vi "intitialize RF synth boards on FPGA 12.5.vi"() -> ()   [LabVIEW 2013]
uses:
  <vilib>/Platform/TimedLoop/XDataNode/timing_clust.ctl
  <vilib>/Platform/TimedLoop/XDataNode/nitl_modes.ctl
  <vilib>/Platform/TimedLoop/XDataNode/wakeup.ctl
  <vilib>/rvi/eio/common/nirviEmuTemplateMethod_errors.vi
  <vilib>/rvi/Emulation/niFpgaSctlEmulationGetInTimedLoop.vi
  <vilib>/rvi/Emulation/niFpgaEmulationReportErrorSimple.vi
  <vilib>/rvi/Emulation/niFpgaGetClockAttributes.vi
  <vilib>/rvi/Emulation/niFpgaCriticalErrorInLSC.vi
  <vilib>/Platform/TimedLoop/XDataNode/XDataNode.xnode
  <vilib>/eio/EIONode/EIONode.xnode
  <vilib>/eio/EIOMethodNode/EIOMethodNode.xnode
  <vilib>/Platform/TimedLoop/XDataNode/XDNodeRunTimeDep.lvlib
panel:
  in  "OSK Bd 1":bool
  in  "Reset Bd 1":bool
  in  "PMODE":bool
  in  "RD":bool
  in  "Address":u8 format="%02x"
  in  "Data BD 1":u8 format="%08b"
  in  "Data BD 2":u8 format="%08b"
  in  "Update Data":bool
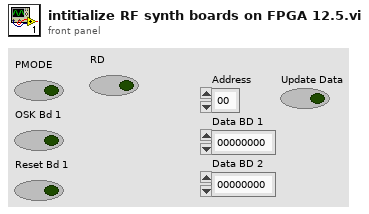
[diagram p1: front panel]
types:
  T1 = typedef "XDNodeRunTimeDep.lvlib/timing_clust.ctl" = cluster{"Expected End [f-1]":u64, "Actual End [f-1]":u64, "Finished Late? [f-1]":bool, "Expected End [i-1]":u64, "Actual End [i-1]":u64, "Finished Late? [i-1]":bool, "Expected Start [i]":u64, "Actual Start [i]":u64, "Expected Start [f]":u64, "Actual Start [f]":u64, "Source Name":string, "Structure Name":string, "Period":i64, "Deadline":i64, "Offset":i64, "Start":i64, "Priority":i32, "Timeout":i32, "Mode":T2, "Wakeup Reason":T3, "Error":errorcluster, "Source Type":string, "Secondary Source Type":string, "Global End Time":u64, "Global Start Time":u64, "Frame Duration":u64, "Iteration Duration":u64, "Assigned CPU":i32, "I/O Scan Engine Mode":u32}
  T2 = typedef "XDNodeRunTimeDep.lvlib/nitl_modes.ctl" = enum32{"No Change", "Process missed periods, maintain original phase", "Discard missed periods, maintain original phase", "Process missed periods, ignore original phase", "Discard missed periods, ignore original phase"}
  T3 = typedef "XDNodeRunTimeDep.lvlib/wakeup.ctl" = enum32{"Normal", "Aborted", "Asynchronous wakeup", "Timing source error", "Timed loop error", "Timeout"}
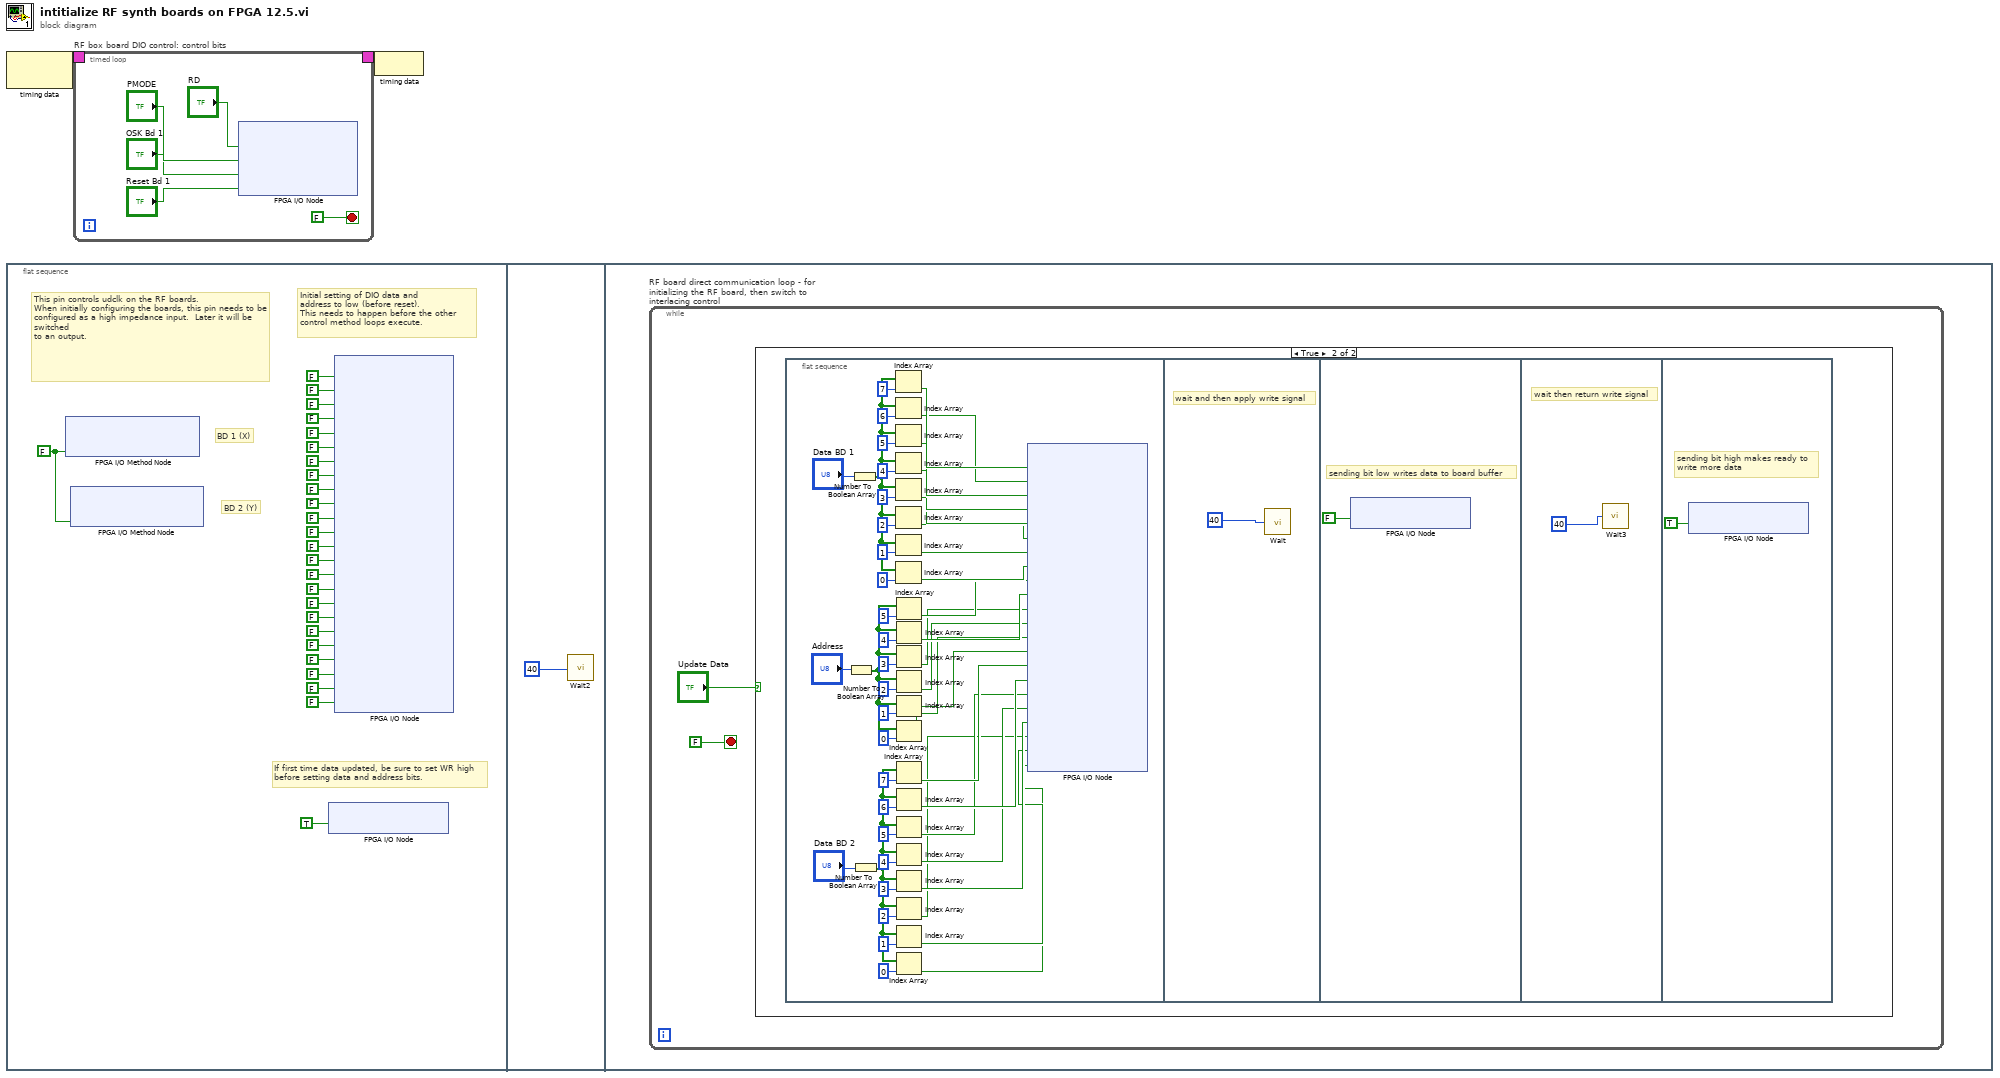
[diagram p0: block diagram]
diagram:
  n1 = node-c288() -> (w2:T1)  [unwired: 1 in]
  n2 = flat-sequence {
    frame #0 {
      w4 = FALSE ("Enable")
      # "If first time data updated, be sure to set WR high\nbefore setting data and address bits."
      # "BD 2 (Y)"
      # "BD 1 (X)"
      # "This pin controls udclk on the RF boards.\nWhen initially configuring the boards, this pin needs to be\nconfigured as a high impedance input.  Later it will be switched\nto an output."
      # "Initial setting of DIO data and \naddress to low (before reset).  \nThis needs to happen before the other\ncontrol method loops execute."
      n3 = xnode "FPGA I/O Method Node"("Enable"=w4) -> ()  [unwired: 1 in, 1 out]
      n4 = xnode "FPGA I/O Method Node"("Enable"=w4) -> ()  [unwired: 1 in, 1 out]
      n5 = xnode "FPGA I/O Node"("Connector1/DIO15"=TRUE) -> ()  [unwired: 1 in, 1 out]
      n6 = xnode "FPGA I/O Node"("Connector1/DIO0"=FALSE, "Connector1/DIO1"=FALSE, "Connector1/DIO2"=FALSE, "Connector1/DIO3"=FALSE, "Connector1/DIO4"=FALSE, "Connector1/DIO5"=FALSE, "Connector1/DIO6"=FALSE, "Connector1/DIO7"=FALSE, "Connector1/DIO8"=FALSE, "Connector1/DIO9"=FALSE, "Connector1/DIO10"=FALSE, "Connector1/DIO11"=FALSE, "Connector1/DIO12"=FALSE, "Connector1/DIO13"=FALSE, "Connector1/DIO15"=FALSE, "Connector1/DIO20"=FALSE, "Connector1/DIO21"=FALSE, "Connector1/DIO22"=FALSE, "Connector1/DIO23"=FALSE, "Connector1/DIO24"=FALSE, "Connector1/DIO25"=FALSE, "Connector1/DIO26"=FALSE, "Connector1/DIO27"=FALSE, "Connector1/DIO14"=FALSE) -> ()  [unwired: 24 in, 24 out]
    }
    frame #1 {
      n7 = call "Wait2"("Count(Ticks)"=u8 40 ("DO Delay 3 (Ticks)")) -> ()  [unwired: 1 out]
    }
    frame #2 {
      n8 = while "RF board direct communication loop - for initializing the RF board, then switch to interlacing control" {
        stop <- FALSE stop-if-true
        n9 = case shown="True" "Update Data" {
          frame False {
          }
          frame True {
            n10 = flat-sequence {
              frame #0 {
                n11 = Number To Boolean Array(number="Address") -> (Boolean array=w78:bool[])
                n12 = Number To Boolean Array(number="Data BD 1") -> (Boolean array=w79:bool[])
                n13 = Number To Boolean Array(number="Data BD 2") -> (Boolean array=w48:bool[])
                n14 = Index Array(array=w79, index=7) -> (element=w63:bool)
                n15 = Index Array(array=w79, index=6) -> (element=w62:bool)
                n16 = Index Array(array=w79, index=5) -> (element=w61:bool)
                n17 = Index Array(array=w79, index=4) -> (element=w60:bool)
                n18 = Index Array(array=w79, index=3) -> (element=w59:bool)
                n19 = Index Array(array=w79, index=2) -> (element=w58:bool)
                n20 = Index Array(array=w79, index=1) -> (element=w57:bool)
                n21 = Index Array(array=w79, index=0) -> (element=w56:bool)
                n22 = Index Array(array=w78, index=5) -> (element=w55:bool)
                n23 = Index Array(array=w78, index=4) -> (element=w54:bool)
                n24 = Index Array(array=w78, index=3) -> (element=w53:bool)
                n25 = Index Array(array=w78, index=2) -> (element=w52:bool)
                n26 = Index Array(array=w78, index=1) -> (element=w51:bool)
                n27 = Index Array(array=w78, index=0) -> (element=w50:bool)
                n28 = Index Array(array=w48, index=7) -> (element=w39:bool)
                n29 = Index Array(array=w48, index=6) -> (element=w38:bool)
                n30 = Index Array(array=w48, index=5) -> (element=w37:bool)
                n31 = Index Array(array=w48, index=4) -> (element=w36:bool)
                n32 = Index Array(array=w48, index=3) -> (element=w35:bool)
                n33 = Index Array(array=w48, index=2) -> (element=w34:bool)
                n34 = Index Array(array=w48, index=1) -> (element=w33:bool)
                n35 = Index Array(array=w48, index=0) -> (element=w32:bool)
                n36 = xnode "FPGA I/O Node"("Connector1/DIO0"=w63, "Connector1/DIO1"=w62, "Connector1/DIO2"=w61, "Connector1/DIO3"=w60, "Connector1/DIO4"=w59, "Connector1/DIO5"=w58, "Connector1/DIO6"=w57, "Connector1/DIO7"=w56, "Connector1/DIO8"=w55, "Connector1/DIO9"=w54, "Connector1/DIO10"=w53, "Connector1/DIO11"=w52, "Connector1/DIO12"=w51, "Connector1/DIO13"=w50, "Connector1/DIO20"=w39, "Connector1/DIO21"=w38, "Connector1/DIO22"=w37, "Connector1/DIO23"=w36, "Connector1/DIO24"=w35, "Connector1/DIO25"=w34, "Connector1/DIO26"=w33, "Connector1/DIO27"=w32) -> ()  [unwired: 22 in, 22 out]
              }
              frame #1 {
                # "wait and then apply write signal"
                n37 = call "Wait"("Count(Ticks)"=u8 40 ("DO Delay 1 (Ticks)")) -> ()  [unwired: 1 out]
              }
              frame #2 {
                # "sending bit low writes data to board buffer"
                n38 = xnode "FPGA I/O Node"("Connector1/DIO15"=FALSE) -> ()  [unwired: 1 in, 1 out]
              }
              frame #3 {
                # "wait then return write signal"
                n39 = call "Wait3"("Count(Ticks)"=u8 40 ("DO Delay 2 (Ticks)")) -> ()  [unwired: 1 out]
              }
              frame #4 {
                # "sending bit high makes ready to\nwrite more data"
                n40 = xnode "FPGA I/O Node"("Connector1/DIO15"=TRUE) -> ()  [unwired: 1 in, 1 out]
              }
            }
          }
        }
      }
    }
  }
  n41 = timed-loop "RF box board DIO control: control bits" {
    timing: w2 -> [_]
    timing-out: [_] -> w1
    stop <- FALSE stop-if-true
    n42 = xnode "FPGA I/O Node"("Connector1/DIO16"="RD", "Connector1/DIO17"="PMODE", "Connector1/DIO18"="OSK Bd 1", "Connector1/DIO19"="Reset Bd 1") -> ()  [unwired: 4 in, 4 out]
  }
  n43 = node-c288(w1) -> ()
